vi "fraction to pulses 2.vi"(10 "fractions":dbl[](array[numeric])=[0.0001, 0.2, 0.49, 0.8, 0.9, 0.99, 0.999, 0.0, 0.0, 0.0, 0.0, 0.0, 0.2, 0.0, 0.0, 0.0]) -> (0 "error out":dbl[](array[numeric])=[0.0001, 0.2, 0.49, 0.8, 0.9, 0.99, 0.999], 1 "switch state":bool[](array[boolean]), 2 "pulses per cycle":u32[](array[numeric]), 3 "pulses on":u32[](array[numeric]), 4 "cycle length (s)":dbl[](array[numeric]), 5 "minimum pulse time (ms) 2":u32)   [LabVIEW 2012]
panel:
  out "Array 3":dbl[](array[numeric])
  out "Array 2":dbl[](array[numeric])
  out "Array":dbl[](array[numeric])
  in  "minimum pulse time (ms)":u32=50
  in  "minimum cycle time (ms)":u32=1000
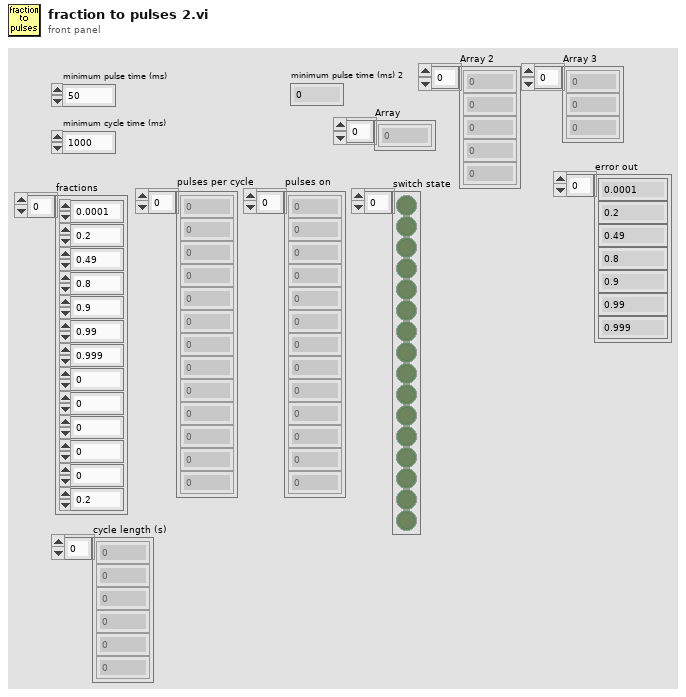
[diagram p1: front panel]
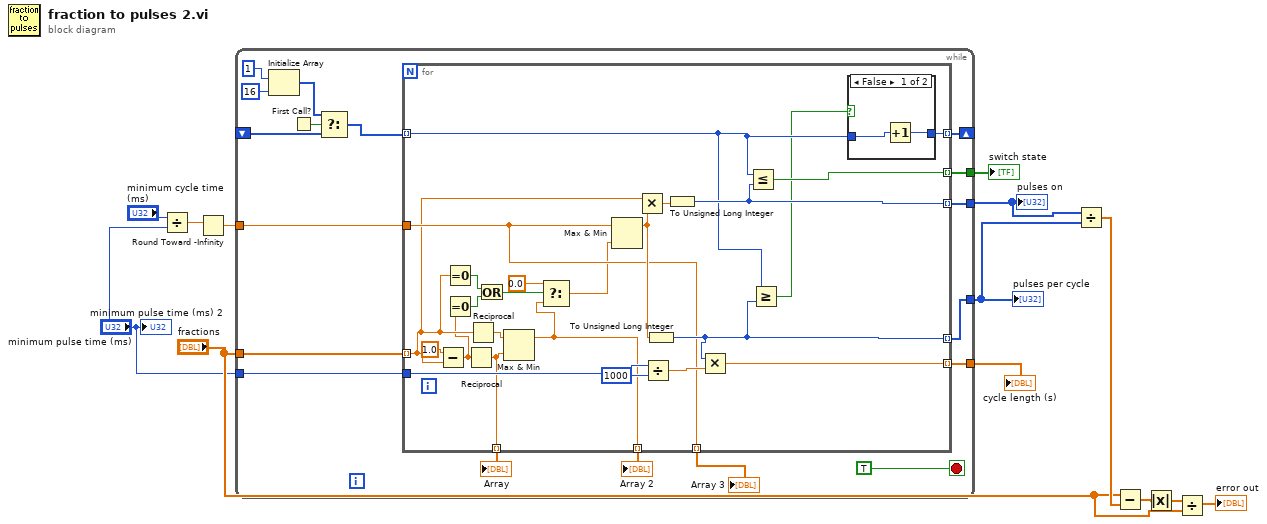
[diagram p0: block diagram]
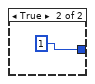
[diagram p2: hidden frame]
diagram:
  n1 = Divide(x="minimum cycle time (ms)", y="minimum pulse time (ms)") -> (x/y=w12:dbl)
  n2 = Round Toward -Infinity(1:w12) -> (0:w6:dbl)
  n3 = while {
    tunnel: "fractions" -> [w31]
    tunnel: w6 -> [w30]
    tunnel: [w29] -> w5
    tunnel: [w28] -> w4
    shift-right: [w26] -> _
    shift-left: _ -> [w24]
    tunnel: [w25] -> w3
    tunnel: "minimum pulse time (ms)" -> [w21]
    tunnel: [w20] -> w1
    stop <- TRUE stop-if-true
    n4 = Initialize Array(1, 16 ("dimension size")) -> (w17:i32[])
    n5 = First Call?() -> (First Call?: T/F=w22:bool)
    n6 = Select(t=w17, s=w22, f=w24) -> (s? t:f=w23:i32[])
    n7 = for {
      tunnel: w31 -> [w39] mode=indexing
      tunnel: [w46] -> w29 mode=indexing
      tunnel: [w51] -> w28 mode=indexing
      tunnel: w30 -> [w40]
      tunnel: [w50] -> w25 mode=indexing
      tunnel: [w49] -> w26 mode=indexing
      tunnel: w23 -> [w48] mode=indexing
      tunnel: w21 -> [w45]
      tunnel: [w44] -> w20 mode=indexing
      tunnel: [w41] -> w16 mode=indexing
      tunnel: [w33] -> w15 mode=indexing
      tunnel: [w40] -> w14 mode=indexing
      n8 = Subtract(x=1.0, y=w39) -> (x-y=w38:dbl)
      n9 = Equal To 0?(x=w39) -> (x = 0?=w36:bool)
      n10 = Equal To 0?(x=w38) -> (x = 0?=w37:bool)
      n11 = Reciprocal(x=w38) -> (1/x=w41:dbl)
      n12 = Reciprocal(x=w39) -> (1/x=w54:dbl)
      n13 = Or(x=w36, y=w37) -> (x .or. y?=w35:bool)
      n14 = Max & Min(x=w54, y=w41) -> (max(x,y)=w33:dbl)  [unwired: 1 out]
      n15 = Select(t=0.0, s=w35, f=w33) -> (s? t:f=w32:dbl)
      n16 = Max & Min(x=w40, y=w32) -> (max(x,y)=w53:dbl)  [unwired: 1 out]
      n17 = Multiply(x=w39, y=w53) -> (x*y=w52:dbl)
      n18 = Divide(x=w45, y=u32 1000) -> (x/y=w43:dbl)
      n19 = To Unsigned Long Integer(number=w53) -> (unsigned 32bit integer=w46:u32)
      n20 = To Unsigned Long Integer(number=w52) -> (unsigned 32bit integer=w51:u32)
      n21 = Multiply(x=w46, y=w43) -> (x*y=w44:dbl)
      n22 = Less Or Equal?(x=w48, y=w51) -> (x <= y?=w50:bool)
      n23 = Greater Or Equal?(x=w48, y=w46) -> (x >= y?=w47:bool)
      n24 = case shown="False" w47 {
        tunnel: [w57 1] -> w49
        tunnel: w48 -> [w56 _]
        frame False {
          n25 = Increment(x=w56) -> (x+1=w57:i32)
        }
        frame True {
        }
      }
    }
    "Array" <- w16
    "Array 2" <- w15
    "Array 3" <- w14
  }
  "pulses per cycle" <- w5
  "pulses on" <- w4
  "switch state" <- w3
  "cycle length (s)" <- w1
  n26 = Divide(x=w4, y=w5) -> (x/y=w11:dbl[])
  n27 = Subtract(x="fractions", y=w11) -> (x-y=w10:dbl[])
  n28 = Absolute Value(x=w10) -> (abs(x)=w7:dbl[])
  n29 = Divide(x=w7, y="fractions") -> (x/y=→"error out":dbl[])
  "minimum pulse time (ms) 2" <- "minimum pulse time (ms)"
